vi "DO Write.vi"(8 "error in (no error)":errorcluster, 9 "data":u8 format="%x", 11 "Data In":T1) -> (0 "error out":errorcluster, 3 "Data Out":T1)   [LabVIEW 2014]
uses:
  controls/Data1.ctl
  controls/Payjson.ctl
  <vilib>/NI Modbus.llb/MB Ethernet Master Query Write Multiple Coils (poly).vi
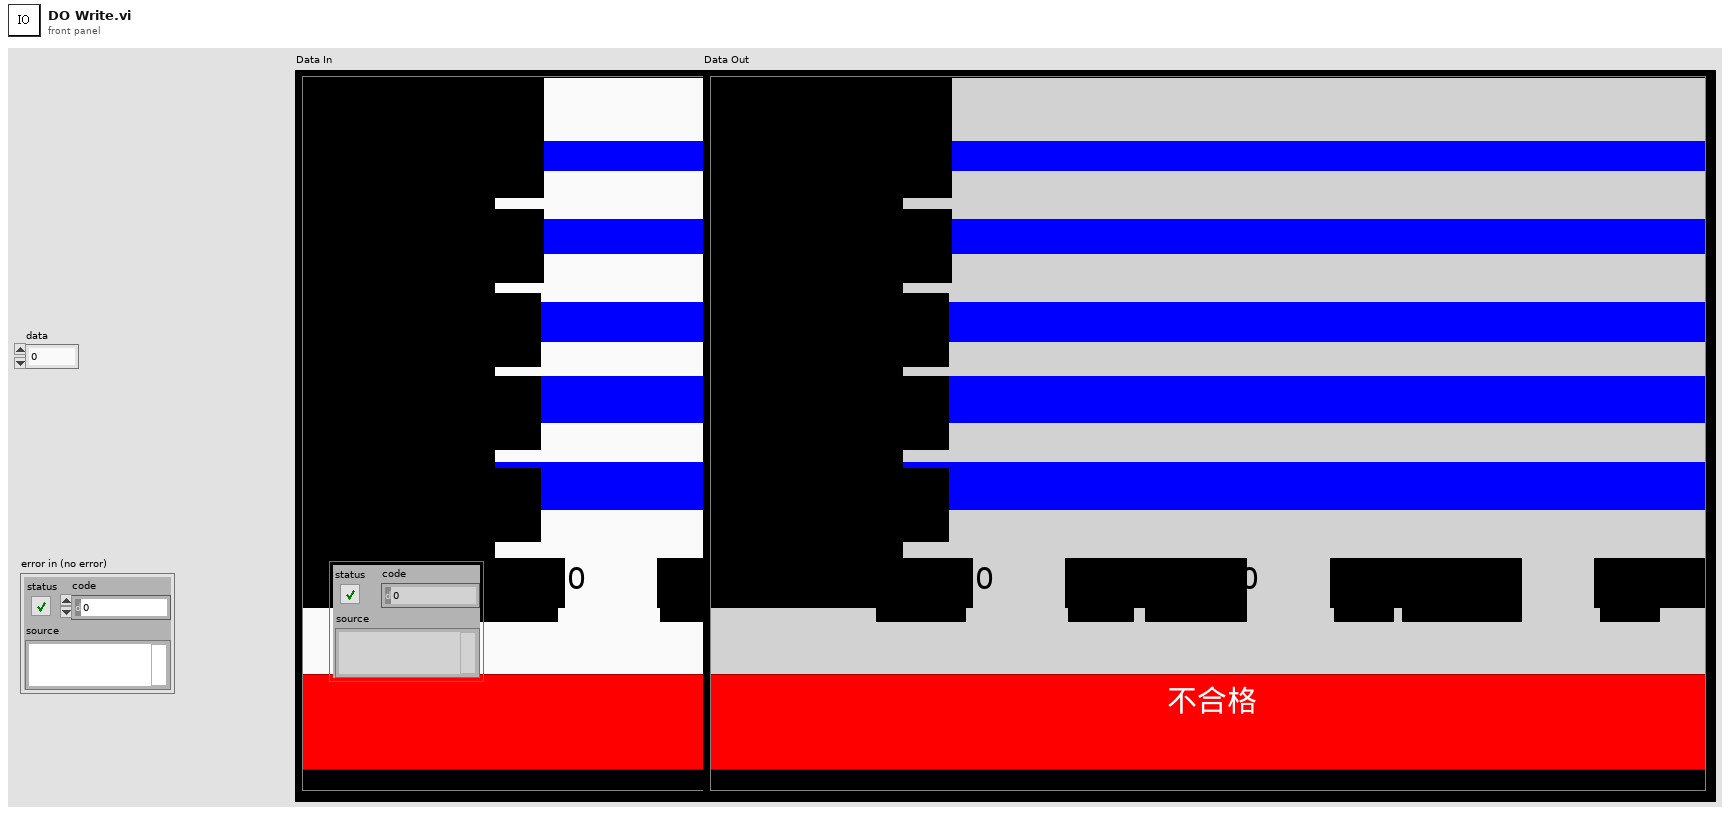
[diagram p1: front panel]
types:
  T1 = typedef "Data1.ctl" = cluster{"Date":string, "BarCode1":string, "BarCode2":string, "BarCode3":string, "Message":string, "OK Count":u16, "NG Count":u16, "Total Count":u16, "ModelData":string[][], "OK&NG":bool, "COM1":refnum<visa-resource-name>, "COM2":refnum<visa-resource-name>, "IO":i32, "Time":u32, "TCP":refnum<k5>, "TCP 2":refnum<k5>, "COM1 2":refnum<visa-resource-name>, "CheckNum":string, "BarCode1_1":string, "BarCode2_1":string, "BarCode3_1":string, "日期":string, "機種":string, "機號":string, "商品條碼1":string, "OK_1":string, "OK":string, "NG":string, "NG_1":string, "Total":string, "Total_1":string, "ClaerTime":u32, "Pjson":T2, "LotNo":string[], "CheckParsArray":string[], "BarCode4":string, "BarCode4_1":string, "商品條碼2":string, "BarCode5":string, "BarCode5_1":string, "商品條碼3":string, "ReScanNG":i32, "NGTimeCT":u32}
  T2 = typedef "Payjson.ctl" = cluster{"DEPT":string, "LINE":string, "STANO":string, "WORKNO":string, "PRODSN":string, "COMPNTID":string, "COMPNTLOT":string, "COMPNTSN":string, "USEDQTY":i16, "OPDATE":string, "OPUSER":string, "RECVDATE":string, "MMODU":string}[]
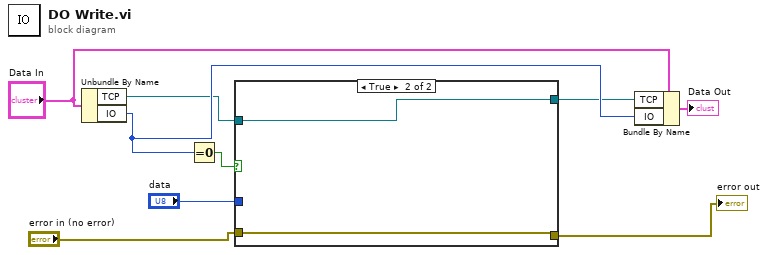
[diagram p0: block diagram]
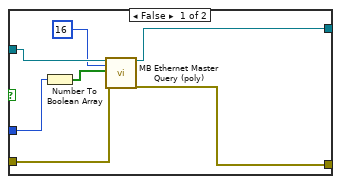
[diagram p2: hidden frame]
diagram:
  n1 = Unbundle By Name("Data In") -> ("TCP"=w6:refnum<k5>, "IO"=w7:i32)
  n2 = Equal To 0?(x=w7) -> (x = 0?=w3:bool)
  n3 = case shown="True" w3 {
    tunnel: w6 -> [w14 w18]
    tunnel: [w13 w18] -> w5
    tunnel: "data" -> [w16 _]
    tunnel: "error in (no error)" -> [w12 w17]
    tunnel: [w11 w17] -> w1
    frame False {
      n4 = Number To Boolean Array(number=w16) -> (Boolean array=w15:bool[])
      n5 = call-poly <vilib>:"MB Ethernet Master Query (poly).vi"("TCP Connection Refnum in"=w14, "Starting Address"=u16 16, "Coils"=w15, "error in"=w12) -> ("TCP Connection Refnum (dup)"=w13:refnum<k5>, "error out"=w11:errorcluster)  [unwired: 13 in, 1 out]
    }
    frame True {
    }
  }
  "error out" <- w1
  n6 = Bundle By Name(cluster="Data In", "TCP"=w5, "IO"=w7) -> (→"Data Out":T1)
